vi "Peer to Peer - 12.8GB Host.vi"() -> ()   [LabVIEW 2023]
uses:
  <vilib>/userDefined/High Color/nirio_resource_hc.ctl
  <vilib>/userDefined/niP2PState.ctl
  <vilib>/FPGAPlugInAG/PXIe-7915/niLvFpga_Open_PXIe-7915.vi
  <vilib>/FPGAPlugInAG/PXIe-7915/niLvFpga_Download_PXIe-7915.vi
  <vilib>/FPGAPlugInAG/PXIe-7915/niLvFpga_Run_PXIe-7915.vi
  <vilib>/FPGAPlugInAG/PXIe-7915/niLvFpga_P2PGetEndpoint_PXIe-7915.vi
  <vilib>/Utility/error.llb/Error Cluster From Error Code.vi
  <vilib>/rvi/errors/niLvFpgaAdjustHostInterfaceError.vi
  <vilib>/FPGAPlugInAG/PXIe-7915/niLvFpga_Close_PXIe-7915.vi
  <vilib>/rvi/interface/nirviOpenFPGA/nirviOpenFPGA.xnode
  <vilib>/rvi/interface/nirviMethod/nirviMethod.xnode
  <vilib>/rvi/interface/nirviReadWriteControl/nirviReadWriteControl.xnode
  <vilib>/rvi/interface/nirviCloseFPGA/nirviCloseFPGA.xnode
  <resource>/objmgr/PeerToPeerStream.rc
  <vilib>/rvi/errors/niLvFpgaMergeErrorWithErrorCode.vi
  NiFpgaLv.dll
  FPGA Bitfiles/P2P_W_7915_12.8GB.lvbitx
  FPGA Bitfiles/P2P_R_PXIe-5785_KU060_12.8GB.lvbitx
  <vilib>/FPGAPlugInAG/PXIe-5785 (KU060)/niLvFpga_Open_PXIe-5785 (KU060).vi
  <vilib>/FPGAPlugInAG/PXIe-5785 (KU060)/niLvFpga_Download_PXIe-5785 (KU060).vi
  <vilib>/FPGAPlugInAG/PXIe-5785 (KU060)/niLvFpga_Run_PXIe-5785 (KU060).vi
  <vilib>/FPGAPlugInAG/PXIe-5785 (KU060)/niLvFpga_P2PGetEndpoint_PXIe-5785 (KU060).vi
  <vilib>/FPGAPlugInAG/PXIe-5785 (KU060)/niLvFpga_Close_PXIe-5785 (KU060).vi
panel:
  out "Data":T1
  out "Stream State":T2
  in  "Reader":T3="RIO1"
  in  "Writer":T3="RIO0"
  out "Transfer Rate (MB/s)":dbl format="%.3f"
  out "Data Valid?":bool
  in  "stop":bool
  in  "Enable":bool
  in  "Flush And Disable":bool
  # "This example shows how to setup and configure a peer to \npeer stream between two PXIe FlexRIO boards. There is a \npeer to peer stream created between the writer and reader \ndevice and once it is enabled, the writer will write a counter \nvalue to the reader. The reader will validate the received\ndata against it's own counter to ensure they match. In \naddition, this example measures throughput of the stream."
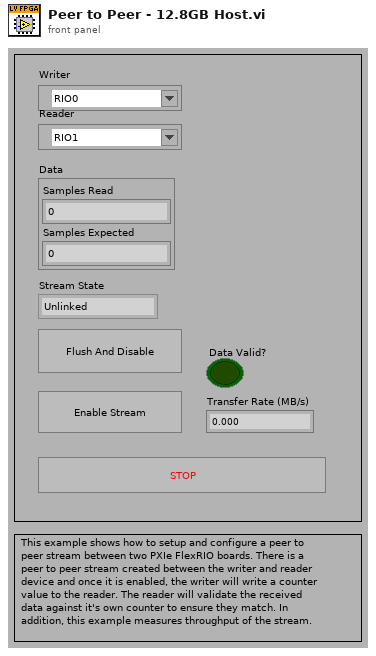
[diagram p1: front panel]
types:
  T1 = cluster{"Samples Read":u64, "Samples Expected":u64}
  T2 = typedef "niP2PState.ctl" = enum32{"Unlinked", "Disabled", "Enabled", "Flushing"}
  T3 = typedef "nirio_resource_hc.ctl" = tag
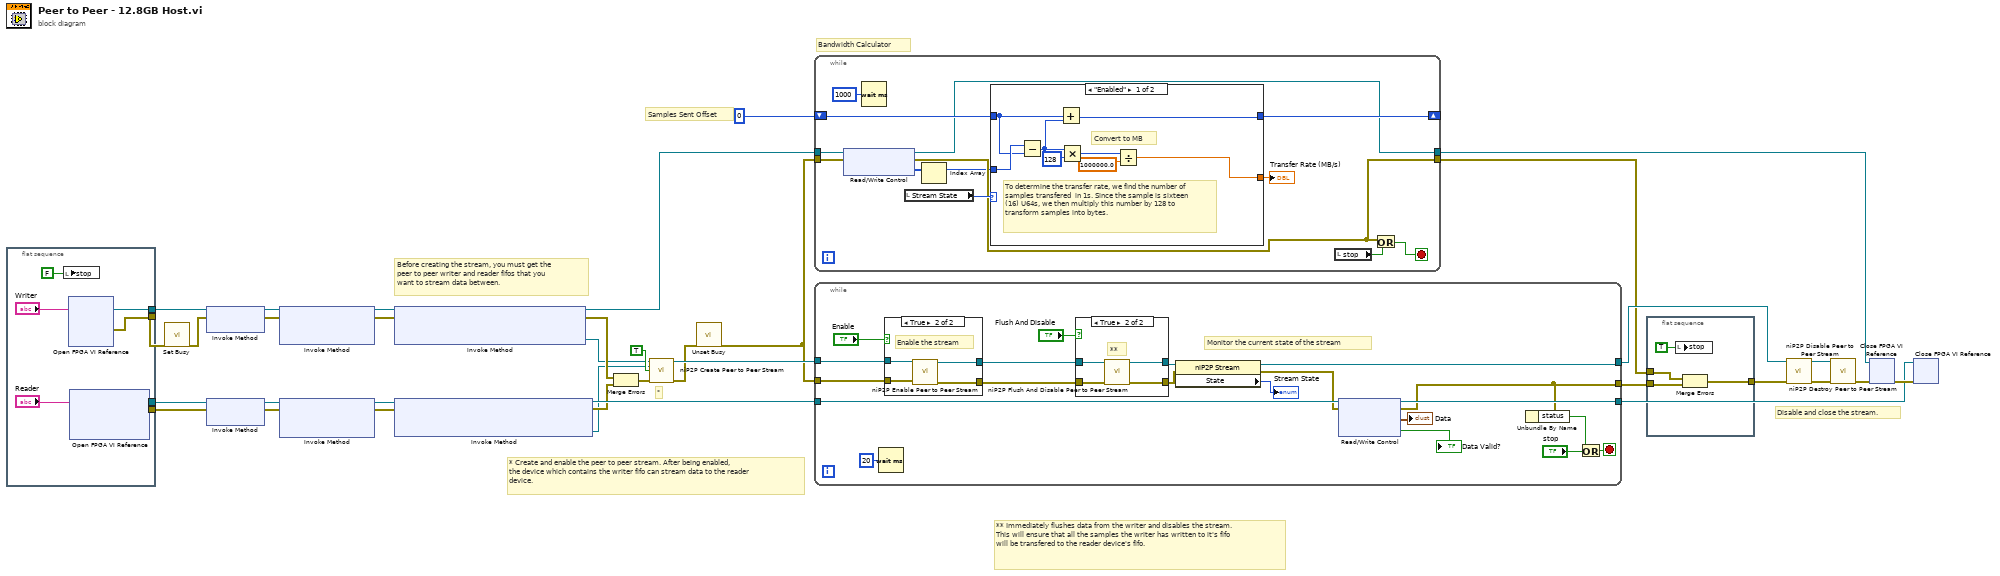
[diagram p0: block diagram]
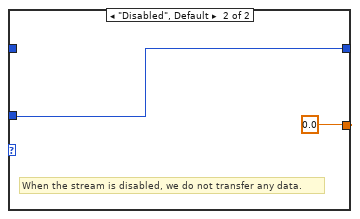
[diagram p2: hidden frame]
diagram:
  # "Bandwidth Calculator"
  # "Samples Sent Offset"
  # "** Immediately flushes data from the writer and disables the stream. \nThis will ensure that all the samples the writer has written to it's fifo \nwill be transfered to the reader device's fifo."
  # "Disable and close the stream."
  # "*"
  # "* Create and enable the peer to peer stream. After being enabled, \nthe device which contains the writer fifo can stream data to the reader\ndevice."
  # "Before creating the stream, you must get the \npeer to peer writer and reader fifos that you \nwant to stream data between."
  n1 = flat-sequence {
    tunnel: [w42] -> w14
    tunnel: [w41] -> w13
    tunnel: [w40] -> w6
    tunnel: [w39] -> w5
    frame #0 {
      n2 = local write "stop"(FALSE ("stop")) -> ()
      n3 = xnode "Open FPGA VI Reference"("resource name"="Writer") -> ("FPGA VI Reference Out"=w42:refnum<k20>, "error out"=w41:errorcluster)  [unwired: 1 in]
      n4 = xnode "Open FPGA VI Reference"("resource name"="Reader") -> ("FPGA VI Reference Out"=w40:refnum<k20>, "error out"=w39:errorcluster)  [unwired: 1 in]
    }
  }
  n5 = call <vilib>:"Set Busy.vi"("error in (no error)"=w13) -> ("error out"=w2:errorcluster)  [unwired: 9 in, 1 out]
  n6 = xnode "Invoke Method"("FPGA VI Reference In"=w14, "error in"=w2) -> ("FPGA VI Reference Out"=w12:refnum<k20>, "error out"=w11:errorcluster)
  n7 = xnode "Invoke Method"("FPGA VI Reference In"=w6, "error in"=w5) -> ("FPGA VI Reference Out"=w8:refnum<k20>, "error out"=w7:errorcluster)
  n8 = xnode "Invoke Method"("FPGA VI Reference In"=w12, "error in"=w11) -> ("FPGA VI Reference Out"=w10:refnum<k20>, "error out"=w9:errorcluster)  [unwired: 1 in]
  n9 = xnode "Invoke Method"("FPGA VI Reference In"=w8, "error in"=w7) -> ("FPGA VI Reference Out"=w4:refnum<k20>, "error out"=w3:errorcluster)  [unwired: 1 in]
  n10 = xnode "Invoke Method"("FPGA VI Reference In"=w10, "error in"=w9) -> ("FPGA VI Reference Out"=w18:refnum<k20>, "error out"=w17:errorcluster, "Writer"=w16:refnum<k20>)
  n11 = xnode "Invoke Method"("FPGA VI Reference In"=w4, "error in"=w3) -> ("FPGA VI Reference Out"=w35:refnum<k20>, "error out"=w34:errorcluster, "Reader"=w15:refnum<k20>)
  n12 = Merge Errors(w17, w34) -> (w33:errorcluster)
  n13 = call <vilib>:"niP2P Create Peer to Peer Stream.vi"("writer"=w16, "reader"=w15, "enable stream (T)"=TRUE, "error in (no error)"=w33) -> ("stream session"=w25:refnum<k20>, "error out"=w24:errorcluster)  [unwired: 10 in]
  n14 = call <vilib>:"Unset Busy.vi"("error in (no error)"=w24) -> ("error out"=w1:errorcluster)  [unwired: 10 in]
  n15 = while {
    tunnel: w18 -> [w49]
    tunnel: w1 -> [w48]
    shift-right: [w50] -> _
    shift-left: u64 0 -> [w51]
    tunnel: [w44] -> w20
    tunnel: [w47] -> w19
    stop <- w53 stop-if-true
    n16 = xnode "Read/Write Control"("FPGA VI Reference In"=w49, "error in"=w48) -> ("FPGA VI Reference Out"=w47:refnum<k20>, "error out"=w44:errorcluster, "Samples Sent"=w45:u64[])
    n17 = Wait (ms)(milliseconds to wait=u32 1000) -> ()  [unwired: 1 out]
    n18 = local read "Stream State"() -> (w52:T2)
    n19 = Index Array(array=w45) -> (element=w43:u64)  [unwired: 1 in]
    n20 = case shown="\"Enabled\"" w52 {
      tunnel: [w59 0.0] -> w55
      tunnel: w51 -> [w58 _]
      tunnel: [w56 w64] -> w50
      tunnel: w43 -> [w63 w64]
      frame "Enabled" {
        # "Convert to MB"
        # "To determine the transfer rate, we find the number of samples transfered  in 1s. Since the sample is sixteen (16) U64s, we then multiply this number by 128 to transform samples into bytes."
        n21 = Subtract(x=w63, y=w58) -> (x-y=w57:u64)
        n22 = Add(x=w58, y=w57) -> (x+y=w56:u64)
        n23 = Multiply(x=w57, y=u64 128) -> (x*y=w62:u64)
        n24 = Divide(x=w62, y=1000000.0) -> (x/y=w59:dbl)
      }
      frame "Disabled", Default {
        # "When the stream is disabled, we do not transfer any data."
      }
    }
    "Transfer Rate (MB/s)" <- w55
    n25 = local read "stop"() -> (w54:bool)
    n26 = Or(x=w44, y=w54) -> (x .or. y?=w53:bool)
  }
  n27 = while {
    tunnel: w25 -> [w83]
    tunnel: w1 -> [w82]
    tunnel: [w73] -> w23
    tunnel: [w69] -> w28
    tunnel: w35 -> [w76]
    tunnel: [w74] -> w31
    stop <- w77 stop-if-true
    # "Monitor the current state of the stream"
    n28 = Wait (ms)(milliseconds to wait=u32 20) -> ()  [unwired: 1 out]
    n29 = case shown="True" "Enable" {
      tunnel: w83 -> [w93 w97]
      tunnel: w82 -> [w92 w96]
      tunnel: [w93 w95] -> w81
      tunnel: [w92 w94] -> w80
      frame False {
      }
      frame True {
        # "Enable the stream"
        n30 = call <vilib>:"niP2P Enable Peer to Peer Stream.vi"("stream session"=w97, "error in (no error)"=w96) -> ("stream session out"=w95:refnum<k20>, "error out"=w94:errorcluster)  [unwired: 12 in]
      }
    }
    n31 = case shown="True" "Flush And Disable" {
      tunnel: w81 -> [w87 w91]
      tunnel: w80 -> [w86 w90]
      tunnel: [w87 w89] -> w71
      tunnel: [w86 w88] -> w70
      frame False {
      }
      frame True {
        # "**"
        n32 = call <vilib>:"niP2P Flush And Disable Peer to Peer Stream.vi"("stream session"=w91, "error in (no error)"=w90) -> ("stream session out"=w89:refnum<k20>, "error out"=w88:errorcluster)  [unwired: 11 in, 1 out]
      }
    }
    n33 = property class="niP2P Stream"(reference=w71, error in=w70) -> (reference out=w69:refnum<k20>, error out=w68:errorcluster, "State"=→"Stream State":T2)
    n34 = xnode "Read/Write Control"("FPGA VI Reference In"=w76, "error in"=w68) -> ("FPGA VI Reference Out"=w74:refnum<k20>, "error out"=w73:errorcluster, "Data"=→"Data":T1, "Data Valid?"=→"Data Valid?":bool)
    n35 = Unbundle By Name(w73) -> ("status"=w78:bool)
    n36 = Or(x=w78, y="stop") -> (x .or. y?=w77:bool)
  }
  n37 = flat-sequence {
    tunnel: w23 -> [w101]
    tunnel: [w100] -> w22
    tunnel: w20 -> [w98]
    frame #0 {
      n38 = local write "stop"(TRUE ("stop")) -> ()
      n39 = Merge Errors(w98, w101) -> (w100:errorcluster)
    }
  }
  n40 = call <vilib>:"niP2P Disable Peer to Peer Stream.vi"("stream session"=w28, "error in (no error)"=w22) -> ("stream session out"=w27:refnum<k20>, "error out"=w26:errorcluster)  [unwired: 12 in]
  n41 = call <vilib>:"niP2P Destroy Peer to Peer Stream.vi"("stream session"=w27, "error in (no error)"=w26) -> ("error out"=w30:errorcluster)  [unwired: 13 in]
  n42 = xnode "Close FPGA VI Reference"("FPGA VI Reference In"=w19, "error in"=w30) -> ("error out"=w32:errorcluster)
  n43 = xnode "Close FPGA VI Reference"("FPGA VI Reference In"=w31, "error in"=w32) -> ()  [unwired: 1 out]
